vi "AIbool.vi"() -> (0 "AIarray":bool[](array[boolean]), 1 "AI?":bool)   [LabVIEW 2013]
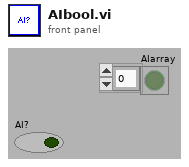
[diagram p1: front panel]
types:
  T1 = cluster{"StageS":i32, "StageL":i32, "data dir":path, "image OD":u16, "contour OD":u16, "point OD":u16, "AOlines":tag[], "AIlines":tag[], "CI lines":tag[], "DO lines":tag[], "AO names":string[], "CI names":string[], "AI names":string[], "DO names":string[]}
  T2 = typedef "LVRectTypeDef.ctl" = cluster{"Left":i16, "Top":i16, "Right":i16, "Bottom":i16}
  T3 = cluster{"Xpixels":i32, "Vxminref":dbl, "Vxmaxref":dbl, "P":dbl, "Ypixels":i32, "Vyminref":dbl, "Vymaxref":dbl, "srate":sgl, "sAOxy":i32, "timeout":dbl, "type":string, "date":string, "time":string, "Colormap":u16, "Drawing Mode":u16, "Scanning Mode":u16, "square pixels":bool, "square matrix":bool, "Xpixels Img":i32, "Vx-min Img":dbl, "VX-max Img":dbl, "Ypixels Img":i32, "Vy-min Img":dbl, "Vy-max Img ":dbl, "Angle Img":dbl, "autoshutter":bool, "finite":bool, "cont":bool, "wavdet":bool, "measpoints":i32, "avpp":i32, "bufferAO":i32, "bufferAI":i32, "starttick":u32, "waveform":path, "Vx-ref":dbl, "Vy-ref":dbl, "refreshrate":dbl, "refreshbuffer":i32, "tt_cycles":i32, "motorref":refnum<k7>, "mirrorswitch":refnum<k7>, "sample mode":i32, "maxbufferAI":i32, "sampletreshold":dbl, "srateAODO":sgl, "bin":sgl, "Pel":sgl, "Angle draw":dbl, "srate Img":sgl, "ROIimg_plotbounds":T2, "auto OD":bool, "ODfilt":u16, "reset AO_DO":bool, "aAI":i32[], "aCI":i32[], "aAO":i32[], "aDO":i32[]}
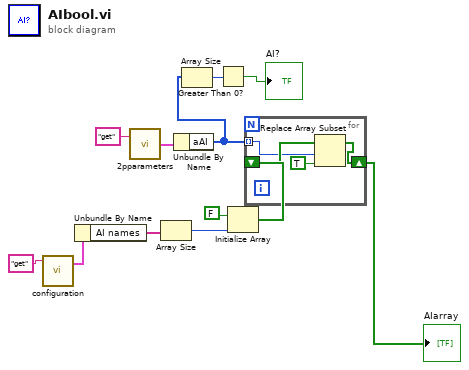
[diagram p0: block diagram]
diagram:
  n1 = call "configuration.vi"("command"="get") -> ("config out"=w9:T1)  [unwired: 2 in, 1 out]
  n2 = Unbundle By Name(w9) -> ("AI names"=w8:string[])
  n3 = call "2pparameters.vi"("command"="get") -> ("params out"=w10:T3)  [unwired: 1 in]
  n4 = Array Size(array=w8) -> (size(s)=w7:i32)
  n5 = Unbundle By Name(w10) -> ("aAI"=w3:i32[])
  n6 = Array Size(array=w3) -> (size(s)=w2:i32)
  n7 = Greater Than 0?(x=w2) -> (x > 0?=→"AI?":bool)
  n8 = Initialize Array(FALSE, w7) -> (w5:bool[])
  n9 = for {
    tunnel: w3 -> [w15] mode=indexing
    shift-right: [w13] -> w4
    shift-left: w5 -> [w16]
    n10 = Replace Array Subset(array=w16, new element=TRUE ("new element/subarray"), index=w15) -> (w13:bool[])
  }
  "AIarray" <- w4
